vi "Read LiDAR Settings.vi"(8 "error in (no error)":errorcluster, 11 "LiDAR in":refnum<class "LiDAR.lvclass">) -> (0 "error out":errorcluster, 2 "LiDAR":T1, 3 "LiDAR out":refnum<class "LiDAR.lvclass">)   [LabVIEW 2018, in "LiDAR.lvlib" / "LiDAR.lvclass"]
uses:
  LiDAR.lvclass
  PPLs/Configuration/Configuration.lvlibp/Configuration.lvclass
  LiDAR.lvclass/LiDAR.ctl
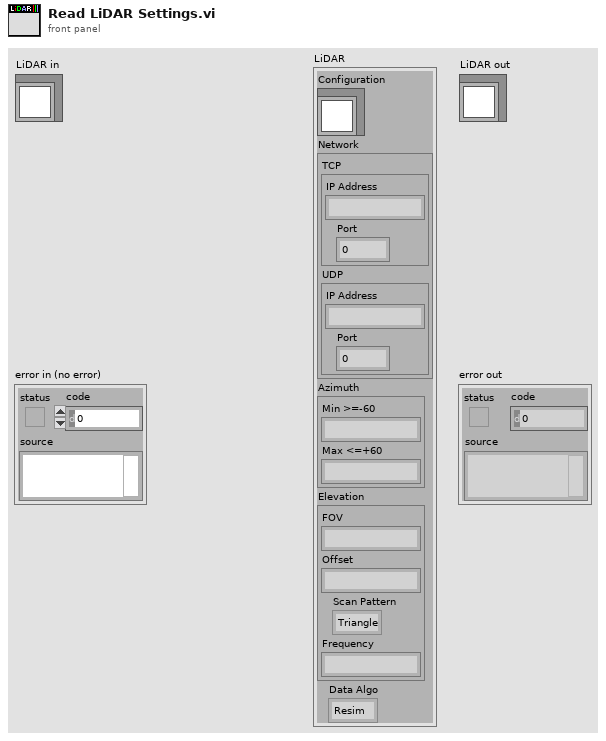
[diagram p1: front panel]
types:
  T1 = cluster{"Configuration":refnum<class "Configuration.lvclass">, "Network":cluster{"TCP":cluster{"IP Address":string, "Port":u16}, "UDP":cluster{"IP Address":string, "Port":u16}}, "Azimuth":cluster{"Min >=-60":string, "Max <=+60":string}, "Elevation":cluster{"FOV":string, "Offset":string, "Scan Pattern":enum16{"Triangle", "Snap"}, "Frequency":string}, "Data Algo":enum16{"Resim", "Point Cloud"}}
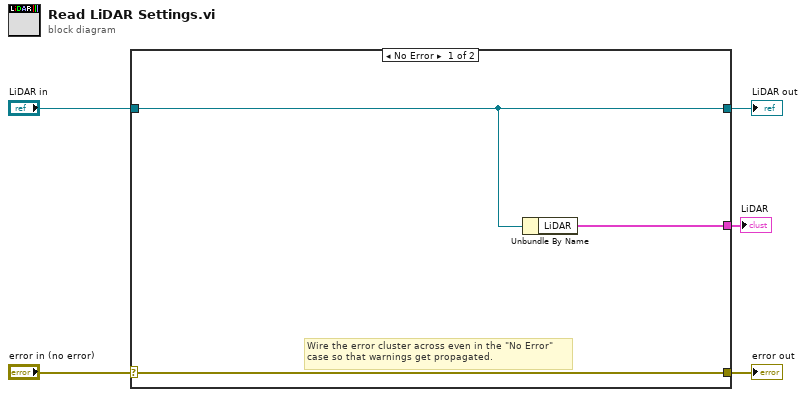
[diagram p0: block diagram]
diagram:
  n1 = case shown="No Error" "error in (no error)" {
    selector: "error in (no error)" -> [w8 w10]
    tunnel: [w8 w10] -> w4
    tunnel: [w7 w9] -> w2
    tunnel: "LiDAR in" -> [w7 w9]
    tunnel: [w6 _] -> w1
    frame No Error {
      # "Wire the error cluster across even in the \"No Error\"\ncase so that warnings get propagated."
      n2 = Unbundle By Name(w7) -> ("LiDAR"=w6:T1)
    }
    frame Error {
    }
  }
  "error out" <- w4
  "LiDAR out" <- w2
  "LiDAR" <- w1
